vi "WavelengthScan.vi"() -> ()   [LabVIEW 2009]
doc: "This VI is an example on how to use the HORIBA Jobin Yvon Monochromator control VIs. To use this VI, press the Run button in LabVIEW.\n\nThe VI will retrieve all configured monochromators from the computer's registry.\n\nSelect the desired monochromator from the Mono ID combo box and press the Connect button to start communications with that device. If the Force Initialization button is enabled, the monochromator will start its automatic calibration routine. If the Force Initialization button is not enabled, the software will keep the monochromator in its current positions.\n\nAfter connecting to the instrument, the VI will retrieve the current positions of all movable motors in the system. This will continue until the Move To Target Position or Stop buttons are pressed.\n\nMove to Target Positions will move the monochromator to the positions entered in the indicators of the VI.\n\nStop will stop running the VI."
panel:
  out "Current Blaze":string
  out "error out":errorcluster
  out "Gratings":dbl[](array[numeric])
  in  "Target Grating":string(combo)
  in  "Target WL":dbl
  in  "Move To\nTarget Positions":bool
  out "Units":string
  in  "Connect":bool
  out "Status":string
  out "Emulating":bool
  out "Initialized":bool
  out "Current UniqueID":string
  in  "Force\nInitialization":bool
  in  "STOP":bool
  out "Current Description":string caption="Description"
  out "Grating Index":i32
  out "Current Grating":dbl
  out "Current WL":dbl
  in  "Mono ID":string(combo)
  # "Setup"
  # "Grating / Wavelength Control"
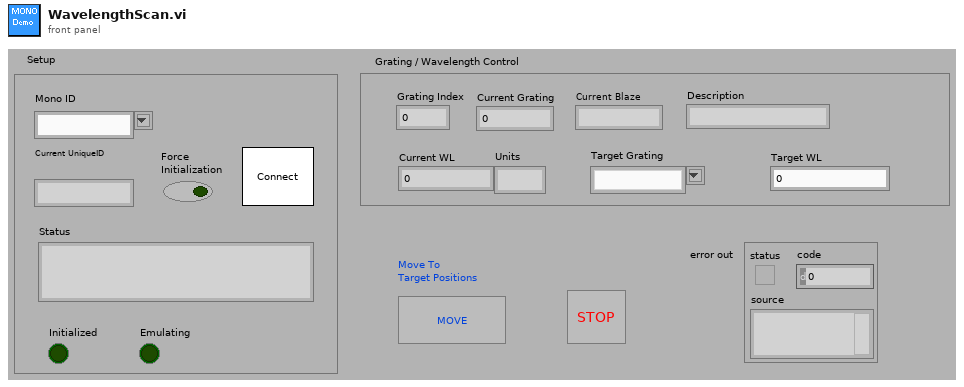
[diagram p1: front panel]
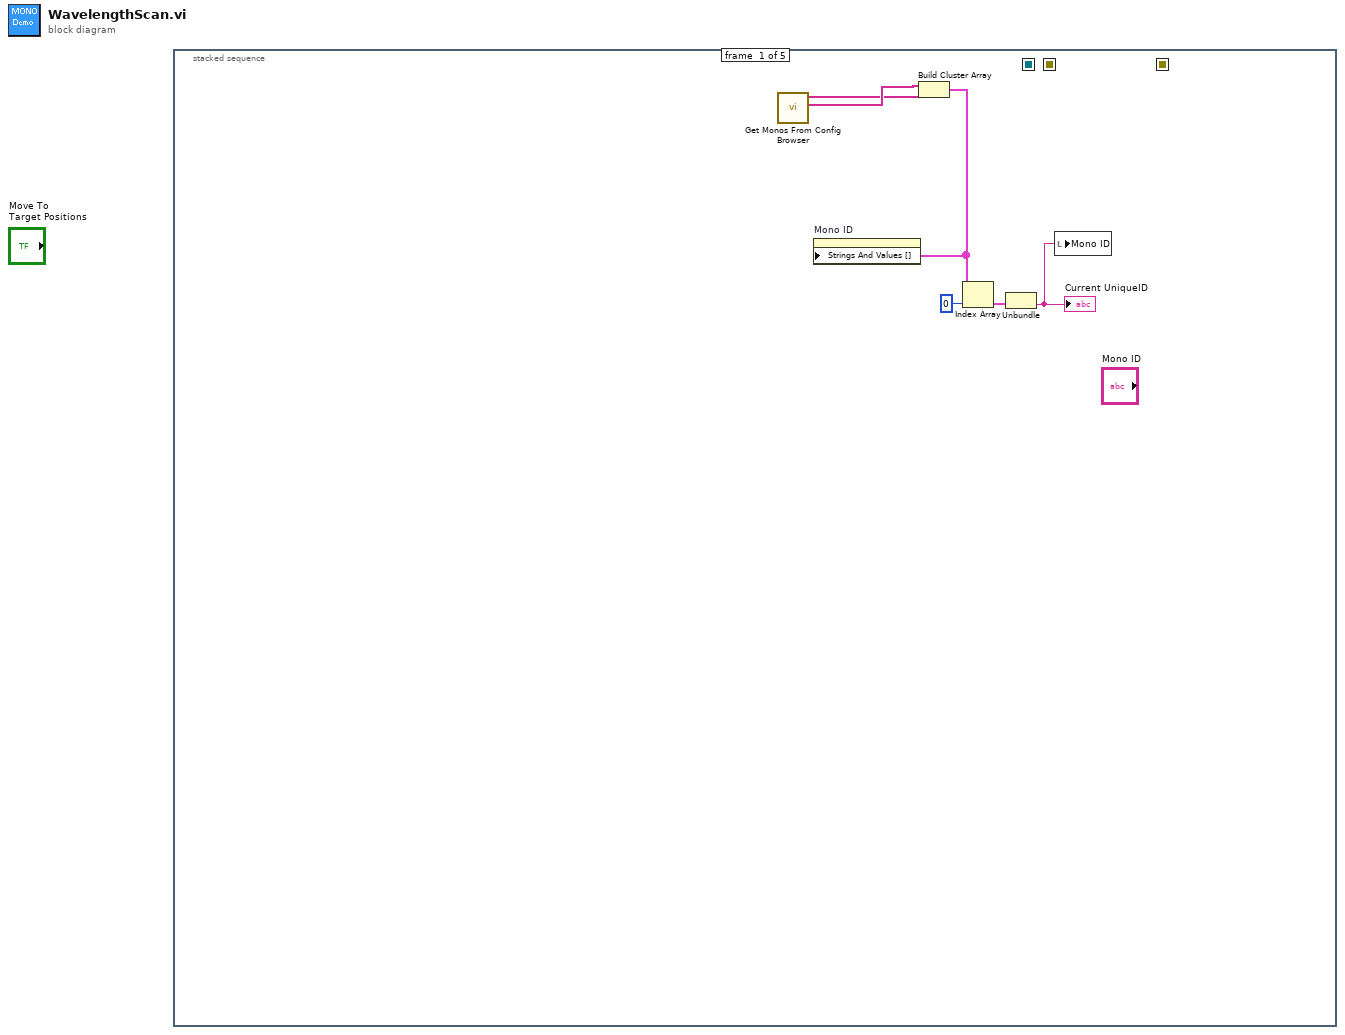
[diagram p0: block diagram]
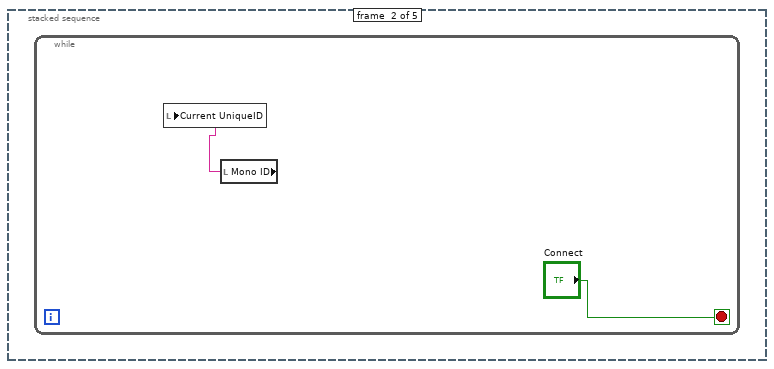
[diagram p2: hidden frame]
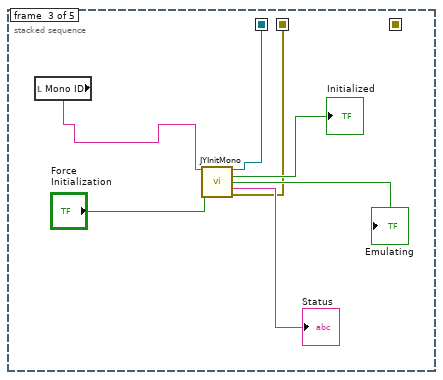
[diagram p3: hidden frame]
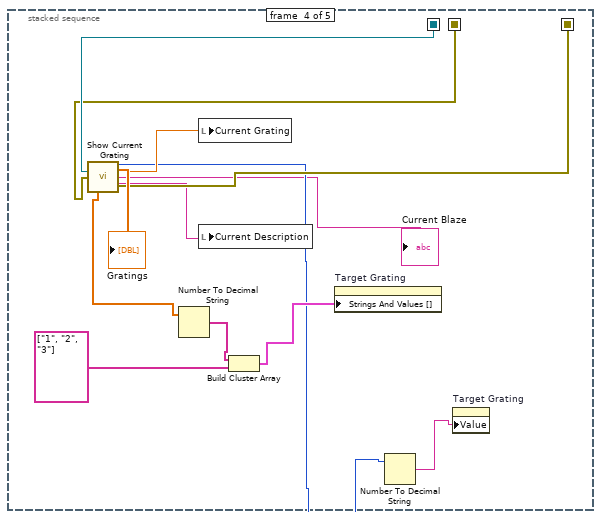
[diagram p4: hidden frame]
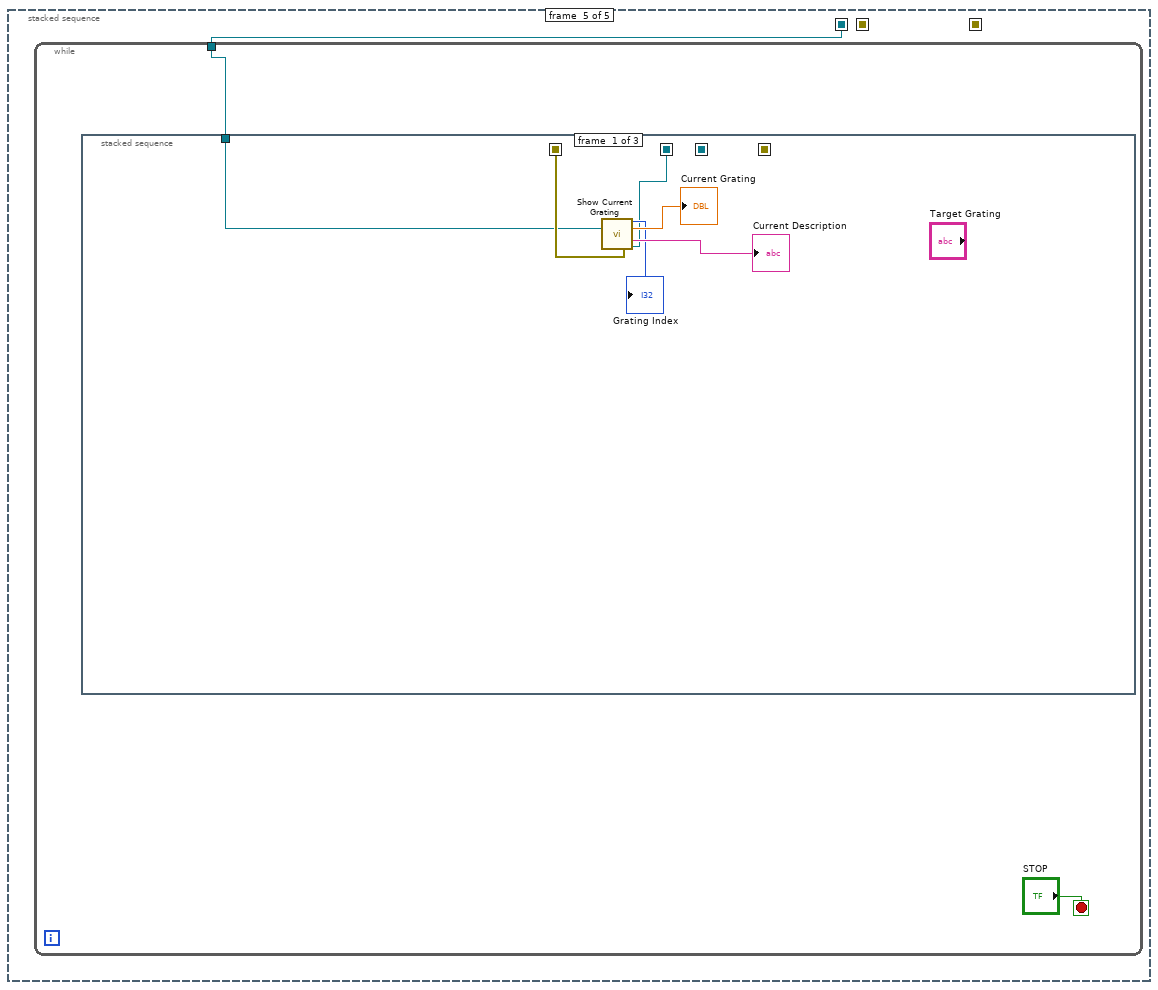
[diagram p5: hidden frame]
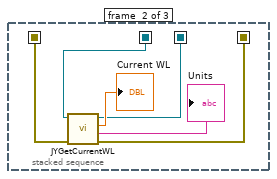
[diagram p6: hidden frame]
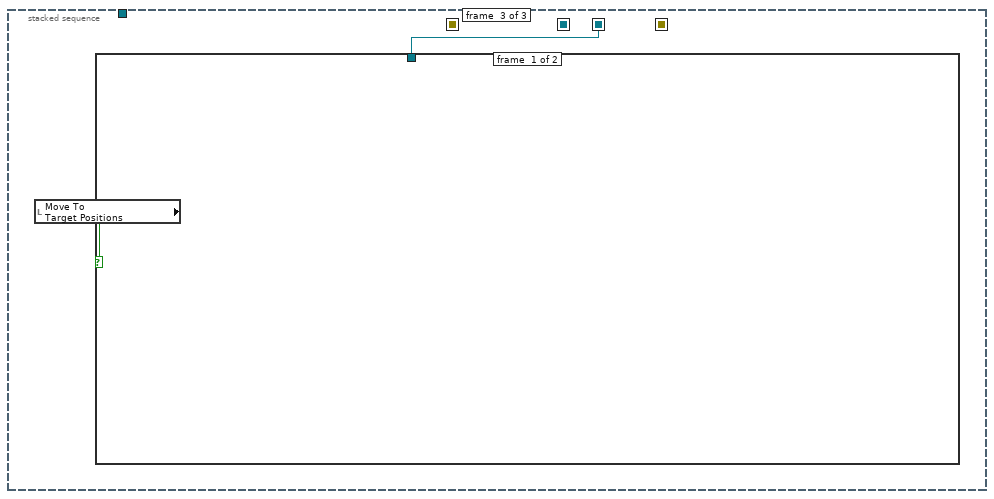
[diagram p7: hidden frame]
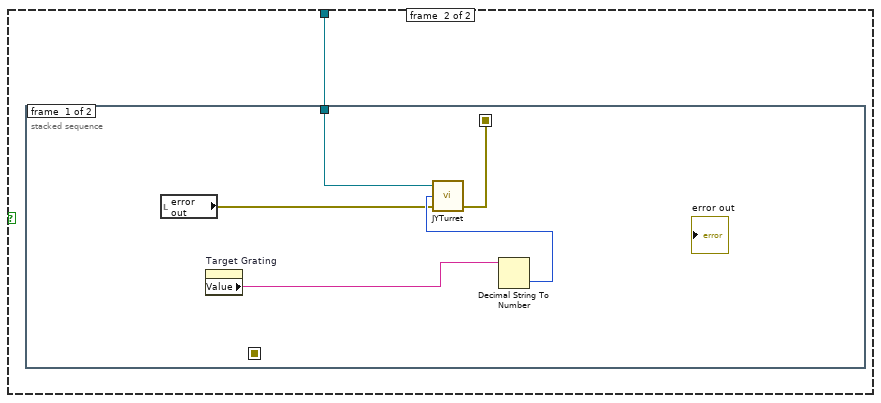
[diagram p8: hidden frame]
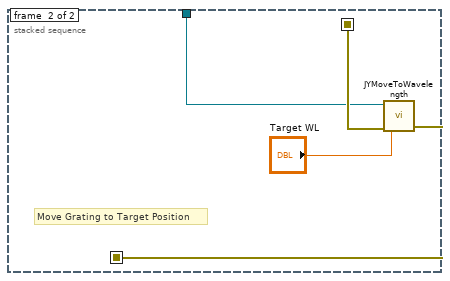
[diagram p9: hidden frame]
diagram:
  n1 = stacked-sequence {
    seq-local: [_ _ w10 _ _] -> [_ _ _ w23 w28]
    seq-local: [_ _ w9 _ _] -> [_ _ _ w22 _]
    seq-local: [_ _ _ w21 _] -> [_ _ _ _ _]
    frame #0 {
      n2 = call "Get Monos From Config Browser.vi"() -> ("UniqueIDs"=w5:string[], "Mono ID"=w6:string[])  [unwired: 3 in, 1 out]
      n3 = Build Cluster Array(w6, w5) -> (w3:cluster{"String":string, "String":string}[])
      n4 = property on="Mono ID" class="CmbBox"("Strings And Values []"=w3) -> ()  [unwired: 2 in, 2 out]
      n5 = Index Array(array=w3, index=0) -> (element=w4:cluster{"String":string, "String":string})
      n6 = Unbundle(w4) -> ("String"=w1:string)  [unwired: 1 out]
      "Current UniqueID" <- w1
      n7 = local write "Mono ID"(w1) -> ()
    }
    frame #1 {
      n8 = while {
        stop <- "Connect" stop-if-true
        n9 = local read "Mono ID"() -> (w7:string)
        n10 = local write "Current UniqueID"(w7) -> ()
      }
    }
    frame #2 {
      n11 = local read "Mono ID"() -> (w14:string)
      n12 = call "JYInitMono.vi"("Unique ID"=w14, "Force Init"="Force\nInitialization") -> ("Refnum out"=w10:refnum<k7>, "Initialized"=→"Initialized":bool, "Emulating"=→"Emulating":bool, "Status"=→"Status":string, "error out"=w9:errorcluster)  [unwired: 9 in]
    }
    frame #3 {
      n13 = call "Show Current Grating.vi"("Refnum in"=w23, "error in (no error)"=w22) -> ("Gratings"=w24:dbl[], "Grating Index"=w18:i32, "Current Grating"=w20:dbl, "Current Blaze"=→"Current Blaze":string, "Current Description"=w17:string, "error out"=w21:errorcluster)  [unwired: 5 in, 3 out]
      "Gratings" <- w24
      n14 = Number To Decimal String(number=w24) -> (decimal integer string=w26:string[])  [unwired: 1 in]
      n15 = local write "Current Grating"(w20) -> ()
      n16 = local write "Current Description"(w17) -> ()
      n17 = Build Cluster Array(w26, string[] ["1", "2", "3"]) -> (w27:cluster{"Numeric":string, string}[])
      n18 = property on="Target Grating" class="CmbBox"("Strings And Values []"=w27) -> ()  [unwired: 2 in, 2 out]
      n19 = Number To Decimal String(number=w18) -> (decimal integer string=w19:string)  [unwired: 1 in]
      n20 = property on="Target Grating" class="CmbBox"("Value"=w19) -> ()  [unwired: 2 in, 2 out]
    }
    frame #4 {
      n21 = while {
        tunnel: w28 -> [w29]
        stop <- "STOP" stop-if-true
        n22 = stacked-sequence {
          seq-local: [w34 _ _] -> [_ w41 _]
          seq-local: [_ w40 _] -> [_ _ _]
          seq-local: [w31 _ _] -> [_ w38 _]
          seq-local: [_ w37 _] -> [_ _ w43]
          tunnel: w29 -> [w33 _ _]
          frame #0 {
            n23 = call "Show Current Grating.vi"("Refnum in"=w33) -> ("Grating Index"=→"Grating Index":i32, "Current Grating"=→"Current Grating":dbl, "Current Description"=→"Current Description":string, "error out"=w34:errorcluster, "Refnum Out"=w31:refnum<k7>)  [unwired: 6 in, 4 out]
          }
          frame #1 {
            n24 = call "JYGetCurrentWL.vi"("error in (no error)"=w41, "JYMONOLib.IJYMonoReqd"=w38) -> ("error out"=w40:errorcluster, "Units"=→"Units":string, "Current WL"=→"Current WL":dbl, "Mono Refnum Out"=w37:refnum<k7>)  [unwired: 6 in]
          }
          frame #2 {
            n25 = local read "Move To\nTarget Positions"() -> (w44:bool)
            n26 = case shown="True" w44 {
              tunnel: w43 -> [_ w45]
              frame #0 {
              }
              frame #1 {
                n27 = stacked-sequence {
                  seq-local: [w49 _] -> [_ w53]
                  seq-local: [_ w52] -> [_ _]
                  tunnel: w45 -> [w46 w51]
                  frame #0 {
                    n28 = local read "error out"() -> (w47:errorcluster)
                    n29 = property on="Target Grating" class="CmbBox"() -> ("Value"=w48:string)  [unwired: 2 in, 2 out]
                    n30 = Decimal String To Number(string=w48) -> (number=w50:i32)  [unwired: 2 in, 1 out]
                    n31 = call "JYTurret.vi"("error in (no error)"=w47, "Grating Index"=w50, "RefNum In"=w46) -> ("error out"=w49:errorcluster)  [unwired: 2 out]
                  }
                  frame #1 {
                    # "Move Grating to Target Position"
                    n32 = call "JYMoveToWavelength.vi"("error in (no error)"=w53, "Target WL"="Target WL", "RefNum In"=w51) -> ("error out"=w52:errorcluster)  [unwired: 1 in, 2 out]
                  }
                }
              }
            }
          }
        }
      }
    }
  }
